vi "index.vi"(2 "index":i8, 3 "where":T1(ring)) -> (0 "Y":dbl, 1 "X":dbl)   [LabVIEW 2023]
uses:
  Shared variables/position1.vi
  Shared variables/position2.vi
  Shared variables/position3.vi
  Shared variables/Shared variables.lvlib
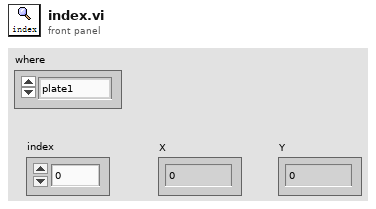
[diagram p1: front panel]
types:
  T1 = enum16{"plate1", "plate2", "plate3", "rinse", "seat"}
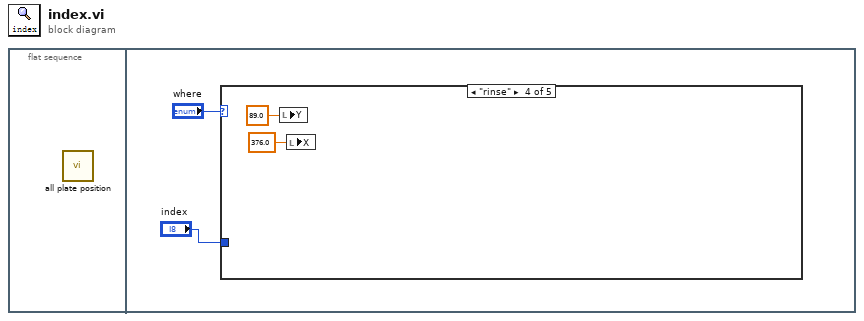
[diagram p0: block diagram]
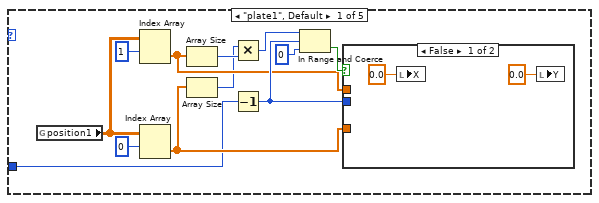
[diagram p2: hidden frame]
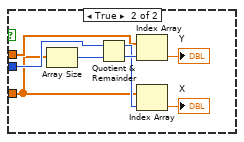
[diagram p3: hidden frame]
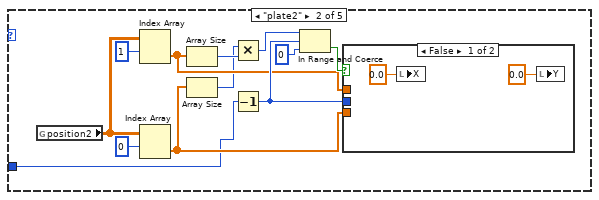
[diagram p4: hidden frame]
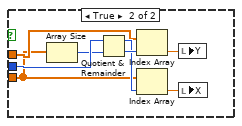
[diagram p5: hidden frame]
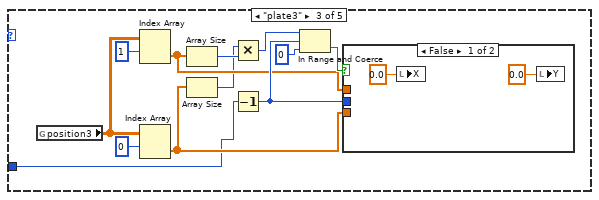
[diagram p6: hidden frame]
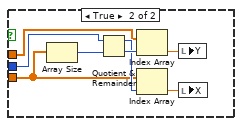
[diagram p7: hidden frame]
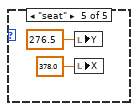
[diagram p8: hidden frame]
diagram:
  n1 = flat-sequence {
    frame #0 {
      n2 = call "all plate position.vi"() -> ()  [unwired: 3 in, 3 out]
    }
    frame #1 {
      n3 = case shown="\"rinse\"" "where" {
        tunnel: "index" -> [w3 w25 w47 _ _]
        frame "plate1", Default {
          n4 = global read "position1.vi" "position1"() -> (w4:dbl[][])
          n5 = Index Array(array=w4, index (row)=1) -> (element=w8:dbl[])  [unwired: 1 in]
          n6 = Index Array(array=w4, index (row)=0) -> (element=w9:dbl[])  [unwired: 1 in]
          n7 = Array Size(array=w8) -> (size(s)=w7:i32)
          n8 = Array Size(array=w9) -> (size(s)=w6:i32)
          n9 = Multiply(x=w6, y=w7) -> (x*y=w5:i32)
          n10 = Decrement(x=w3) -> (x-1=w12:i8)
          n11 = In Range and Coerce(upper limit=w5, x=w12, lower limit=i8 0 ("upper limit")) -> (In Range?=w14:bool)  [unwired: 1 out]
          n12 = case shown="False" w14 {
            tunnel: w12 -> [_ w23]
            tunnel: w8 -> [_ w18]
            tunnel: w9 -> [_ w17]
            frame False {
              n13 = local write "X"(0.0 ("X")) -> ()
              n14 = local write "Y"(0.0 ("Y")) -> ()
            }
            frame True {
              n15 = Array Size(array=w17) -> (size(s)=w19:i32)
              n16 = Quotient & Remainder(x=w23, y=w19) -> (x-y*floor(x/y)=w20:i32, floor(x/y)=w21:i32)
              n17 = Index Array(array=w18, index=w21) -> (element=→"Y":dbl)
              n18 = Index Array(array=w17, index=w20) -> (element=→"X":dbl)
            }
          }
        }
        frame "plate2" {
          n19 = global read "position2.vi" "position2"() -> (w36:dbl[][])
          n20 = Index Array(array=w36, index (row)=1) -> (element=w32:dbl[])  [unwired: 1 in]
          n21 = Index Array(array=w36, index (row)=0) -> (element=w33:dbl[])  [unwired: 1 in]
          n22 = Array Size(array=w32) -> (size(s)=w31:i32)
          n23 = Array Size(array=w33) -> (size(s)=w30:i32)
          n24 = Multiply(x=w30, y=w31) -> (x*y=w29:i32)
          n25 = Decrement(x=w25) -> (x-1=w34:i8)
          n26 = In Range and Coerce(upper limit=w29, x=w34, lower limit=i8 0 ("upper limit")) -> (In Range?=w35:bool)  [unwired: 1 out]
          n27 = case shown="False" w35 {
            tunnel: w34 -> [_ w46]
            tunnel: w32 -> [_ w42]
            tunnel: w33 -> [_ w41]
            frame False {
              n28 = local write "X"(0.0 ("X")) -> ()
              n29 = local write "Y"(0.0 ("Y")) -> ()
            }
            frame True {
              n30 = Array Size(array=w41) -> (size(s)=w43:i32)
              n31 = Quotient & Remainder(x=w46, y=w43) -> (x-y*floor(x/y)=w44:i32, floor(x/y)=w45:i32)
              n32 = Index Array(array=w42, index=w45) -> (element=w40:dbl)
              n33 = Index Array(array=w41, index=w44) -> (element=w39:dbl)
              n34 = local write "Y"(w40) -> ()
              n35 = local write "X"(w39) -> ()
            }
          }
        }
        frame "plate3" {
          n36 = global read "position3.vi" "position3"() -> (w48:dbl[][])
          n37 = Index Array(array=w48, index (row)=1) -> (element=w55:dbl[])  [unwired: 1 in]
          n38 = Index Array(array=w48, index (row)=0) -> (element=w56:dbl[])  [unwired: 1 in]
          n39 = Array Size(array=w55) -> (size(s)=w54:i32)
          n40 = Array Size(array=w56) -> (size(s)=w53:i32)
          n41 = Multiply(x=w53, y=w54) -> (x*y=w52:i32)
          n42 = Decrement(x=w47) -> (x-1=w57:i8)
          n43 = In Range and Coerce(upper limit=w52, x=w57, lower limit=i8 0 ("upper limit")) -> (In Range?=w58:bool)  [unwired: 1 out]
          n44 = case shown="False" w58 {
            tunnel: w57 -> [_ w68]
            tunnel: w55 -> [_ w64]
            tunnel: w56 -> [_ w63]
            frame False {
              n45 = local write "X"(0.0 ("X")) -> ()
              n46 = local write "Y"(0.0 ("Y")) -> ()
            }
            frame True {
              n47 = Array Size(array=w63) -> (size(s)=w65:i32)
              n48 = Quotient & Remainder(x=w68, y=w65) -> (x-y*floor(x/y)=w66:i32, floor(x/y)=w67:i32)
              n49 = Index Array(array=w64, index=w67) -> (element=w62:dbl)
              n50 = Index Array(array=w63, index=w66) -> (element=w61:dbl)
              n51 = local write "Y"(w62) -> ()
              n52 = local write "X"(w61) -> ()
            }
          }
        }
        frame "rinse" {
          n53 = local write "Y"(89.0 ("Y")) -> ()
          n54 = local write "X"(376.0 ("X")) -> ()
        }
        frame "seat" {
          n55 = local write "Y"(276.5 ("Y")) -> ()
          n56 = local write "X"(378.0 ("X")) -> ()
        }
      }
    }
  }
